vi "DELETE Number of Samples.vi"   [LabVIEW 2013]
uses:
  Action.ctl
  Experimental Parameters FGV Selector.ctl
types:
  T1 = typedef "Experimental Parameters FGV Selector.ctl" = enum16{"Number of Samples", "Ramp Rate", "Z Scan Size"}
  T2 = typedef "Action.ctl" = enum16{"GET", "PUT", "DELETE"}
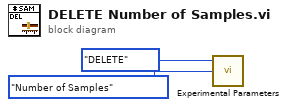
[diagram p0: block diagram]
diagram:
  n1 = call "Experimental Parameters.vi"("Experimental Parameters FGV Selector"=Experimental_Parameters_FGV_Selector."Number of Samples", "Action"=Action."DELETE") -> ()  [unwired: 1 in, 1 out]
